vi "CRYView Global.vi"() -> ()   [LabVIEW 2013]
panel:
  in  "cCurverOutDataList":T1(array[cluster])
  in  "sActiveView":string
  in  "ViewCommand":T2
  out "VIRefCommandQueue":refnum<vi>
  in  "ViewCommandList":T3(array[cluster])
  in  "SetGraphDataList":cluster{"sAction":string, "sData":string}[](array[cluster])
  in  "cBootDATAVIEW":T4
  out "sDefaultGraph":string="XY"
  in  "cBootVIEW":T4
  in  "cCurverOutData":T5
  out "VIRefOuting":refnum<vi>
  in  "cView":T6
  in  "pathViewLog":path
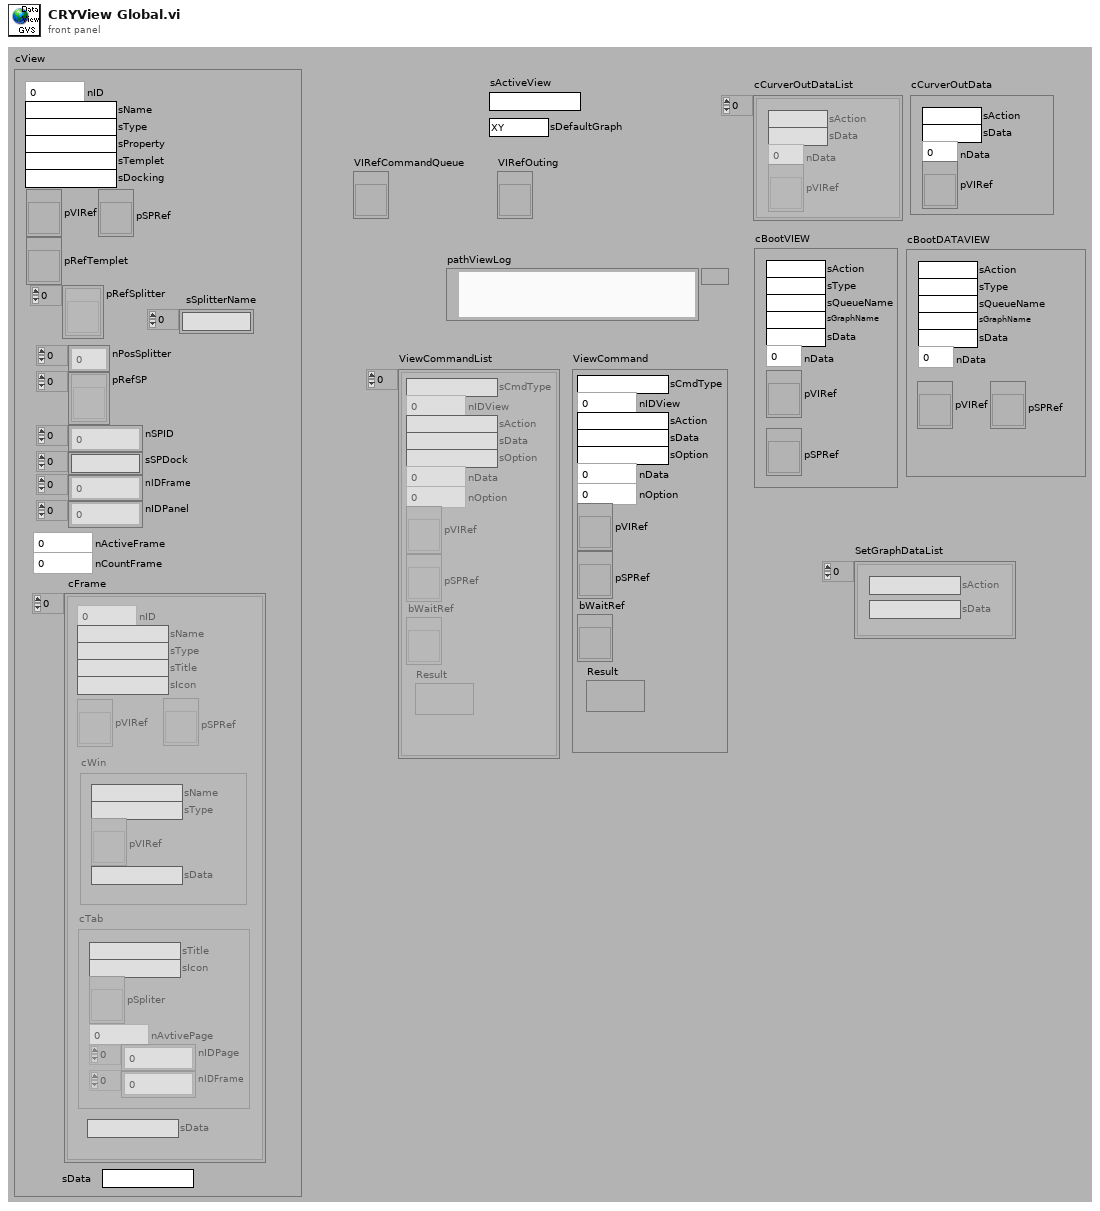
[diagram p1: front panel]
types:
  T1 = cluster{"sAction":string, "sData":string, "nData":i32, "pVIRef":refnum<vi>}[]
  T2 = cluster{"sCmdType":string, "nIDView":i32, "sAction":string, "sData":string, "sOption":string, "nData":i32, "nOption":i32, "pVIRef":refnum<vi>, "pSPRef":refnum<vi>, "bWaitRef":refnum<vi>, "Result":variant}
  T3 = cluster{"sCmdType":string, "nIDView":i32, "sAction":string, "sData":string, "sOption":string, "nData":i32, "nOption":i32, "pVIRef":refnum<vi>, "pSPRef":refnum<vi>, "bWaitRef":refnum<vi>, "Result":variant}[]
  T4 = cluster{"sAction":string, "sType":string, "sQueueName":string, "sGraphName":string, "sData":string, "nData":i32, "pVIRef":refnum<vi>, "pSPRef":refnum<vi>}
  T5 = cluster{"sAction":string, "sData":string, "nData":i32, "pVIRef":refnum<vi>}
  T6 = cluster{"nID":i32, "sName":string, "sType":string, "sProperty":string, "sTemplet":string, "sDocking":string, "pVIRef":refnum<vi>, "pSPRef":refnum<vi>, "pRefTemplet":refnum<vi>, "pRefSplitter":refnum<vi>[], "nPosSplitter":i32[], "pRefSP":refnum<vi>[], "nSPID":i32[], "sSPDock":string[], "nIDFrame":i32[], "nIDPanel":i32[], "nActiveFrame":i32, "nCountFrame":i32, "cFrame":cluster{"nID":i32, "sName":string, "sType":string, "sTitle":string, "sIcon":string, "pVIRef":refnum<vi>, "pSPRef":refnum<vi>, "cWin":cluster{"sName":string, "sType":string, "pVIRef":refnum<vi>, "sData":string}, "cTab":cluster{"sTitle":string, "sIcon":string, "pSpliter":refnum<vi>, "nAvtivePage":i32, "nIDPage":i32[], "nIDFrame":i32[]}, "sData":string}[], "sData":string, "sSplitterName":string[]}
diagram:
